vi "sos uncert 2024.vi"(0 "Temperature / K":dbl=293.15 format="%.4g", 1 "Pressure / Pa":dbl=101325.0 format="%.1f", 2 "Frequency / Hz":dbl, 3 "xw water molar fraction":dbl format="%.6f", 4 "CO2 content (ppm)":dbl=500.0, 5 "Type of air":i32(listbox)=4) -> (6 "heat capacity correction Kc (ppm)":dbl=-1018.6498795005106, 7 "1/2 heat capacity speed correction Kc/2 (ppm)":dbl=-509.3249397502553, 8 "virial correction Kv (ppm)":dbl=586.7080324797198, 9 "1/2 virial speed correction Kv/2 (ppm)":dbl=293.3540162398599, 10 "relaxation correction Kr (ppm)":dbl format="%#.0f", 11 "1/2 relax speed correction Kr/2 (ppm)":dbl, 13 "combined (quadrature sum) relative uncertainty of speed of sound in humid air due to corrections (ppm)":dbl=19.554822241525684 format="%.1f", 14 "DKc/1+Kc (ppm)":dbl=0.25731867133520203 format="%.1f", 15 "DKv/1+Kv (ppm)":dbl=38.85232581171617, 16 "DKr/1+Kr (ppm)":dbl, 17 "1/2 * DKc/1+Kc - heat capacity rel. uncert. contribution to speed of sound (ppm)":dbl=0.12865933566760102 format="%.1f", 18 "1/2 * DKv/1+Kv - virial rel. uncert. contribution to speed of sound (ppm)":dbl=19.426162905858085 format="%.1f", 19 "1/2 * DKr/1+Kr - relaxation rel. uncert. contribution to speed of sound (ppm)":dbl format="%.1g")   [LabVIEW 2016]
panel:
  # "±"
  # "±"
  # "±"
  # "±"
  # "±"
  # "±"
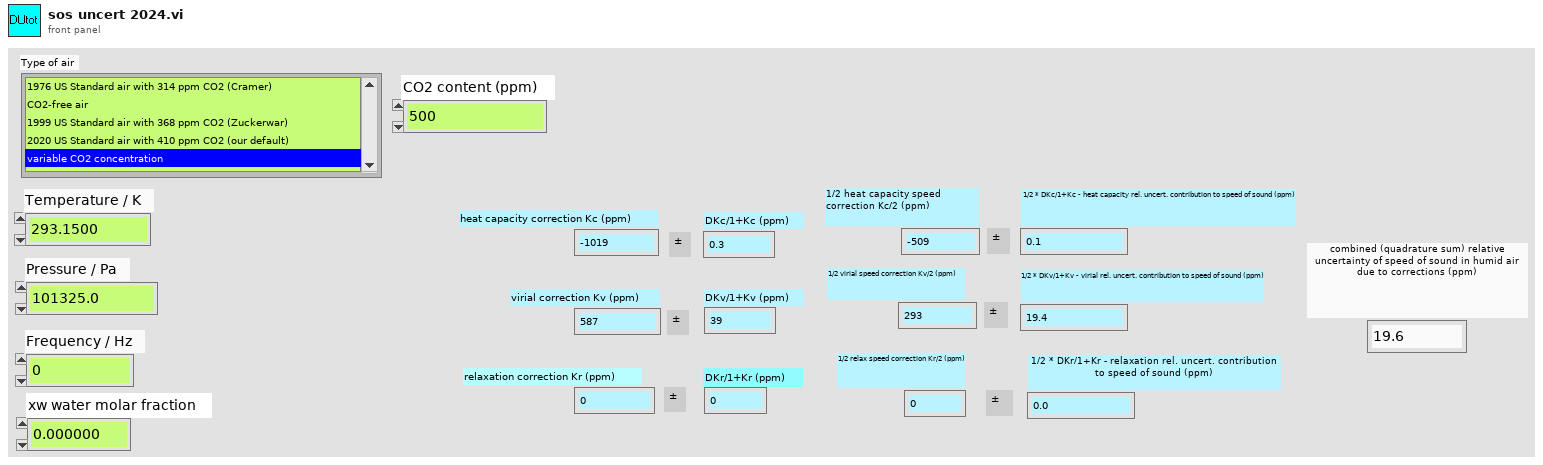
[diagram p1: front panel]
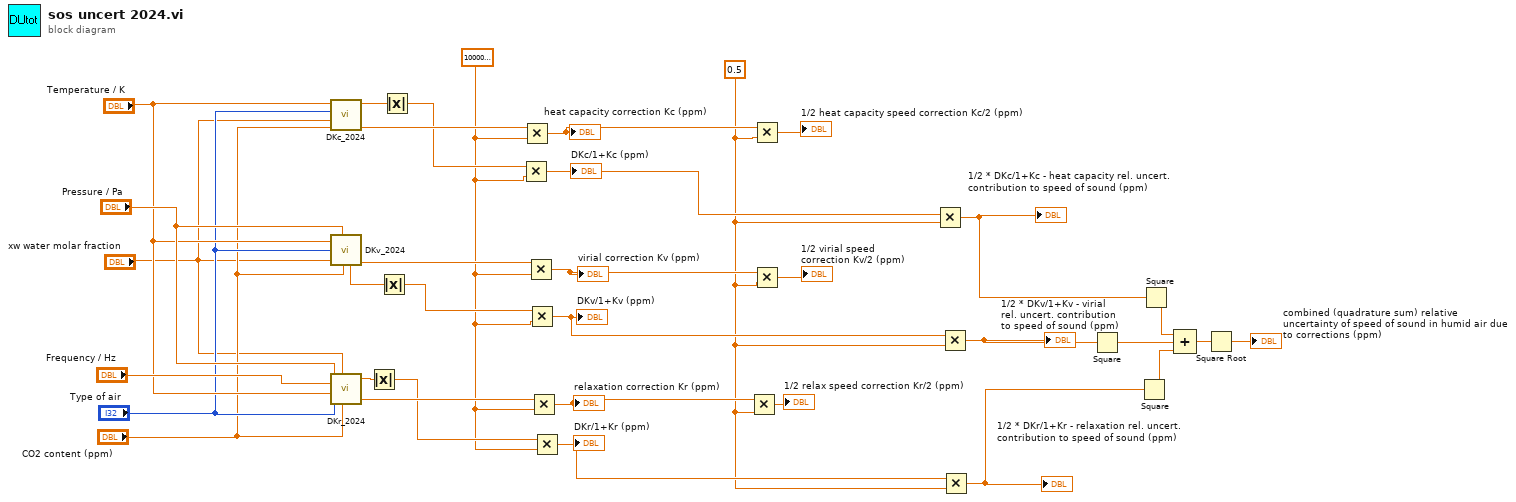
[diagram p0: block diagram]
diagram:
  w15 = 1000000.0 ("y")
  w8 = 0.5 ("x")
  n1 = call "DKc_2024.vi"("Temperature / K"="Temperature / K", "Type of air"="Type of air", "xw water mol. fract."="xw water molar fraction", "CO2 content (ppm)"="CO2 content (ppm)") -> ("DKc/1+Kc"=w22:dbl, "Kc - correzione"=w24:dbl)  [unwired: 3 out]
  n2 = call "DKv_2024.vi"("Temperature [K]"="Temperature / K", "Pressure [Pa]"="Pressure / Pa", "Type of air"="Type of air", "xw molar fraction of water vapor"="xw water molar fraction", "CO2 content (ppm)"="CO2 content (ppm)") -> ("DKv/1+Kv"=w21:dbl, "Kv"=w23:dbl)  [unwired: 4 out]
  n3 = call "DKr_2024.vi"("Pressure / Pa"="Pressure / Pa", "xw mol fract water"="xw water molar fraction", "Frequency / Hz"="Frequency / Hz", "Temperature / K"="Temperature / K", "CO2 content (ppm)"="CO2 content (ppm)", "Type of air"="Type of air") -> ("DKr/1+Kr"=w20:dbl, "Kr"=w19:dbl)  [unwired: 1 out]
  n4 = Absolute Value(x=w20) -> (abs(x)=w16:dbl)
  n5 = Absolute Value(x=w21) -> (abs(x)=w17:dbl)
  n6 = Absolute Value(x=w22) -> (abs(x)=w18:dbl)
  n7 = Multiply(x=w18, y=w15) -> (x*y=w14:dbl)
  "DKc/1+Kc (ppm)" <- w14
  n8 = Multiply(x=w24, y=w15) -> (x*y=w11:dbl)
  "heat capacity correction Kc (ppm)" <- w11
  n9 = Multiply(x=w23, y=w15) -> (x*y=w10:dbl)
  "virial correction Kv (ppm)" <- w10
  n10 = Multiply(x=w17, y=w15) -> (x*y=w13:dbl)
  "DKv/1+Kv (ppm)" <- w13
  n11 = Multiply(x=w19, y=w15) -> (x*y=w9:dbl)
  "relaxation correction Kr (ppm)" <- w9
  n12 = Multiply(x=w16, y=w15) -> (x*y=w12:dbl)
  "DKr/1+Kr (ppm)" <- w12
  n13 = Multiply(x=w9, y=w8) -> (x*y=→"1/2 relax speed correction Kr/2 (ppm)":dbl)
  n14 = Multiply(x=w11, y=w8) -> (x*y=→"1/2 heat capacity speed correction Kc/2 (ppm)":dbl)
  n15 = Multiply(x=w10, y=w8) -> (x*y=→"1/2 virial speed correction Kv/2 (ppm)":dbl)
  n16 = Multiply(x=w14, y=w8) -> (x*y=w27:dbl)
  "1/2 * DKc/1+Kc - heat capacity rel. uncert. contribution to speed of sound (ppm)" <- w27
  n17 = Multiply(x=w13, y=w8) -> (x*y=w26:dbl)
  "1/2 * DKv/1+Kv - virial rel. uncert. contribution to speed of sound (ppm)" <- w26
  n18 = Multiply(x=w12, y=w8) -> (x*y=w25:dbl)
  "1/2 * DKr/1+Kr - relaxation rel. uncert. contribution to speed of sound (ppm)" <- w25
  n19 = Square(x=w26) -> (x^2=w3:dbl)
  n20 = Square(x=w25) -> (x^2=w2:dbl)
  n21 = Square(x=w27) -> (x^2=w4:dbl)
  n22 = Compound Arithmetic op=ADD(w4, w3, w2) -> (w28:dbl)
  n23 = Square Root(x=w28) -> (sqrt(x)=→"combined (quadrature sum) relative uncertainty of speed of sound in humid air due to corrections (ppm)":dbl)
